vi "Msg to Send.vi"(10 "Error":errorcluster) -> (3 "Destroy Msg out":refnum<class "Destroy Msg.lvclass">)   [LabVIEW 2021, in "Destroy.lvlib" / "Destroy Msg.lvclass"]
uses:
  Destroy Msg.lvclass
  Destroy Msg.lvclass/Destroy Msg.ctl
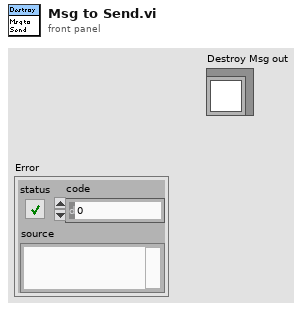
[diagram p1: front panel]
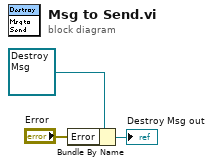
[diagram p0: block diagram]
diagram:
  n1 = Bundle By Name(cluster=refnum<class "Destroy Msg.lvclass"> refnum ("Destroy Msg in"), "Error"="Error") -> (→"Destroy Msg out":refnum<class "Destroy Msg.lvclass">)
